vi "IsArmed.vi"(8 "error in (no error)":errorcluster, 11 "DAQmx Digitizer in":refnum<class "DAQmx Digitizer.lvclass">) -> (0 "error out":errorcluster, 1 "Finished":bool, 2 "Armed":bool, 3 "DAQmx Digitizer out":refnum<class "DAQmx Digitizer.lvclass">, 4 "Availiable Samples":u32)   [LabVIEW 2015, in "DAQmx Digitizer.lvclass"]
uses:
  DAQmx Digitizer.lvclass
  DAQmx Digitizer.lvclass/DAQmx Digitizer.ctl
  <resource>/objmgr/daqmx.rc
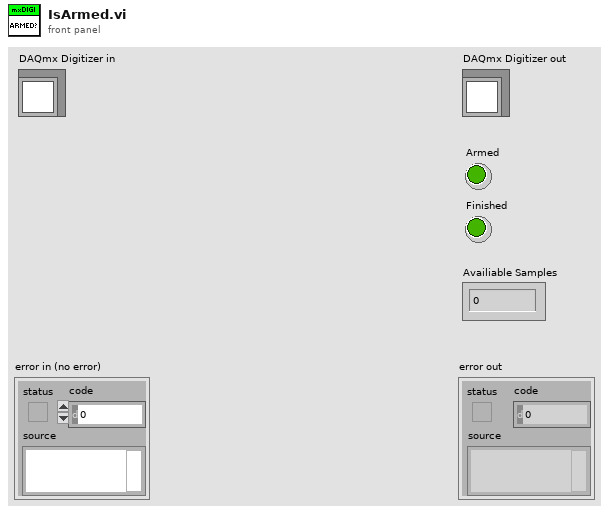
[diagram p1: front panel]
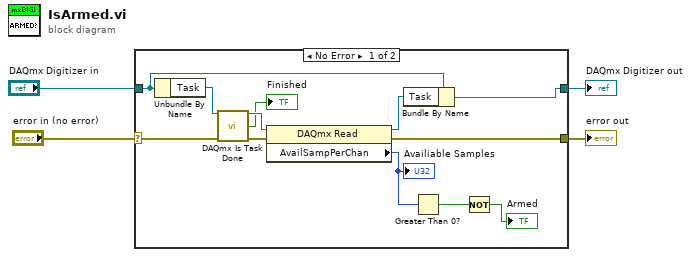
[diagram p0: block diagram]
diagram:
  n1 = case shown="No Error" "error in (no error)" {
    selector: "error in (no error)" -> [w11 w18]
    tunnel: [w10 w18] -> w3
    tunnel: [w9 w17] -> w1
    tunnel: "DAQmx Digitizer in" -> [w13 w17]
    frame No Error {
      n2 = Unbundle By Name(w13) -> ("Task"=w12:refnum<k21>)
      n3 = call <vilib>:"DAQmx Is Task Done.vi"("task/channels in"=w12, "error in"=w11) -> ("task out"=w16:refnum<k21>, "task done?"=→"Finished":bool, "error out"=w15:errorcluster)  [unwired: 11 out]
      n4 = property class="DAQmx Read"(reference=w16, error in=w15) -> (reference out=w8:refnum<k21>, error out=w10:errorcluster, "AvailSampPerChan"=w7:u32)
      "Availiable Samples" <- w7
      n5 = Bundle By Name(cluster=w13, "Task"=w8) -> (w9:refnum<class "DAQmx Digitizer.lvclass">)
      n6 = Greater Than 0?(x=w7) -> (x > 0?=w14:bool)
      n7 = Not(x=w14) -> (.not. x?=→"Armed":bool)
    }
    frame Error {
    }
  }
  "error out" <- w3
  "DAQmx Digitizer out" <- w1
